vi "DriveDist.vi"(8 "error in (no error)":errorcluster, 9 "Timeout":dbl=5.0, 10 "DriveDist":dbl=108.0, 11 "saturation Dist":dbl=0.9) -> (0 "error out":errorcluster)   [LabVIEW 2016]
uses:
  <vilib>/Rock Robotics/WPI/Utilities/WPI_GetSetVariantRefNum.vi
  Robot Global Data.vi
  <vilib>/addons/control/pid/pid.llb/PID (DBL).vi
  <vilib>/Rock Robotics/WPI/RobotDrive/WPI_RobotDriveArcadeDrive_Standard(NoSaturation).vi
  <vilib>/addons/control/pid/NI_PID_pid.lvlib
panel:
  in  "Tolerance":dbl=0.5
  in  "PID gains":T1={"proportional gain (Kc)"=0.2, "integral time (Ti, min)"=0.0, "derivative time (Td, min)"=0.0} {"derivative time (Td, min)" format="%.7f"; "integral time (Ti, min)" format="%.7f"; "proportional gain (Kc)" format="%.3f"}
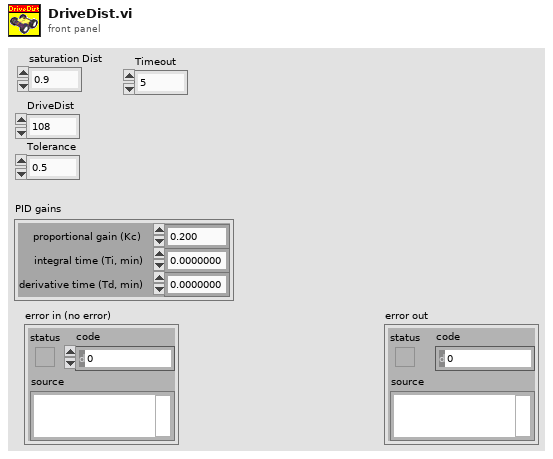
[diagram p1: front panel]
types:
  T1 = cluster{"proportional gain (Kc)":dbl, "integral time (Ti, min)":dbl, "derivative time (Td, min)":dbl}
  T2 = typedef "WPI_RobotDriveDevRef.ctl" = cluster{"DevStatus":errorcluster, "Motors[]":T3[], "Square Inputs":bool, "Max Output":dbl}
  T3 = typedef "WPI_MotorControlDeviceRef.ctl" = cluster{"DeviceStatus":errorcluster, "Type":T4, "PWM":cluster{"PWM Channel":T5, "DeadBand":T6}, "CAN":cluster{"Device Number":u8, "SetOutput VI Ref":variant, "GetOutput VI Ref":variant, "Enable VI Ref":variant, "Disable VI Ref":variant, "Data":variant}, "Invert":bool}
  T4 = typedef "WPI_MotorControlType.ctl" = enum16{"PWM", "CAN"}
  T5 = typedef "FPGA_DIOPWMChannel.ctl" = enum8{"PWM 0", "PWM 1", "PWM 2", "PWM 3", "PWM 4", "PWM 5", "PWM 6", "PWM 7", "PWM 8", "PWM 9", "PWM MXP 0", "PWM MXP 1", "PWM MXP 2", "PWM MXP 3", "PWM MXP 4", "PWM MXP 5", "PWM MXP 6", "PWM MXP 7", "PWM MXP 8", "PWM MXP 9", "Invalid"}
  T6 = typedef "WPI_PWMDeadband.ctl" = cluster{"Name":string, "maxPositivePwm":i32, "minPositivePwm":i32, "centerPwm":i32, "maxNegativePwm":i32, "minNegativePwm":i32, "angularRange":u16}
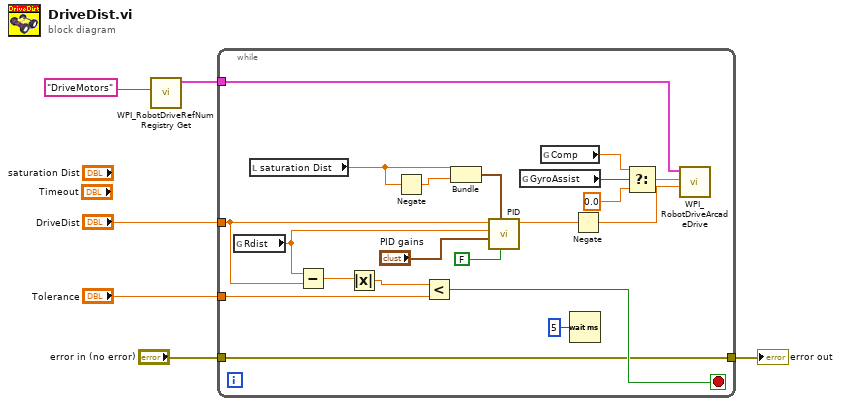
[diagram p0: block diagram]
diagram:
  n1 = call <vilib>:"WPI_RobotDriveRefNum Registry Get.vi"("refnum name"="DriveMotors") -> ("RobotDriveDevRef"=w5:T2)  [unwired: 1 in, 9 out]
  n2 = while {
    tunnel: w5 -> [w20]
    tunnel: "DriveDist" -> [w17]
    tunnel: "Tolerance" -> [w14]
    tunnel: [w12] -> w2
    tunnel: "error in (no error)" -> [w12]
    stop <- w13 stop-if-true
    n3 = global read "Robot Global Data.vi" "Rdist"() -> (w18:dbl)
    n4 = local read "saturation Dist"() -> (w22:dbl)
    n5 = Subtract(x=w18, y=w17) -> (x-y=w16:dbl)
    n6 = Absolute Value(x=w16) -> (abs(x)=w15:dbl)
    n7 = Negate(x=w22) -> (-x=w26:dbl)
    n8 = Less?(x=w15, y=w14) -> (x < y?=w13:bool)
    n9 = Bundle("saturation Dist"=w22, w26) -> (w25:cluster{"saturation Dist":dbl, dbl})  [unwired: 1 out]
    n10 = call-poly <vilib>:"PID.vi"("reinitialize? (F)"=FALSE, "output range"=w25, "PID gains"="PID gains", "process variable"=w18, "setpoint"=w17) -> ("output"=w23:dbl)  [unwired: 1 in, 5 out]
    n11 = global read "Robot Global Data.vi" "GyroAssist"() -> (w7:bool)
    n12 = global read "Robot Global Data.vi" "Comp"() -> (w8:dbl)
    n13 = Wait (ms)(milliseconds to wait=u32 5) -> ()  [unwired: 1 out]
    n14 = Negate(x=w23) -> (-x=w21:dbl)
    n15 = Select(t=w8, s=w7, f=0.0 ("X axis value")) -> (s? t:f=w10:dbl)
    n16 = call-poly <vilib>:"WPI_RobotDriveArcadeDrive.vi"("Y axis value"=w21, "X axis value"=w10, "RobotDriveDevRef"=w20) -> ()  [unwired: 6 in, 3 out]
  }
  "error out" <- w2
